vi "Build Command Frame.vi"(0 "RFFE Extended Command in":refnum<class "RFFE Extended Command.lvclass">, 11 "error in (no error)":errorcluster) -> (4 "RFFE Extended Command out":refnum<class "RFFE Extended Command.lvclass">, 6 "Command Frame":u8[](array[numeric]), 15 "error out":errorcluster)   [LabVIEW 2018, in "MIPI RFFE API.lvlib" / "RFFE Extended Command.lvclass"]
uses:
  RFFE Extended Command.lvclass
  C:/Users/semoore/Projects/mipi-rffe-labview-oop/Command/RFFE Command.lvclass
  Command/RFFE Command.lvclass/RFFE Command.ctl
  Command/Get Slave Address.vi
  Command/Get Command Bits.vi
  Get Byte Count Field Width.vi
  MIPI RFFE API.lvlib
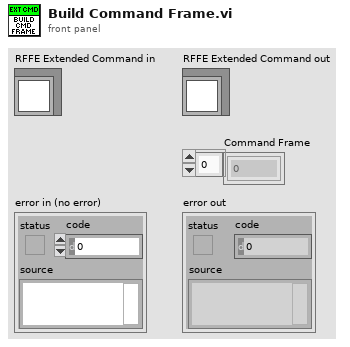
[diagram p1: front panel]
types:
  T1 = typedef "RFFE Commands.lvlib/Slave Address.ctl" = u8
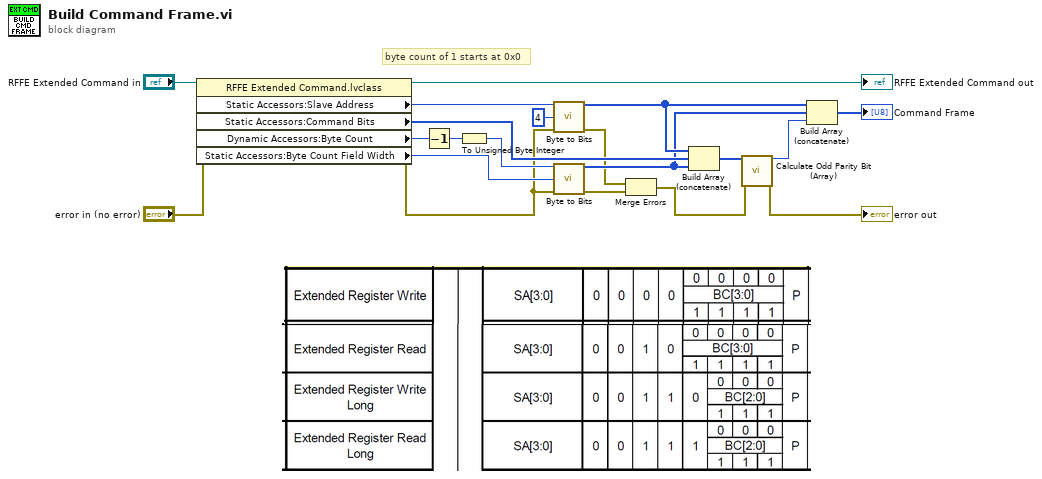
[diagram p0: block diagram]
diagram:
  # "byte count of 1 starts at 0x0"
  n1 = property class="RFFE Extended Command.lvclass"(reference="RFFE Extended Command in", error in="error in (no error)") -> (reference out=→"RFFE Extended Command out":refnum<class "RFFE Extended Command.lvclass">, error out=w6:errorcluster, "Static Accessors:Slave Address"=w9:T1, "Static Accessors:Command Bits"=w8:u8[], "Dynamic Accessors:Byte Count"=w1:i32, "Static Accessors:Byte Count Field Width"=w14:i32)
  n2 = Decrement(x=w1) -> (x-1=w2:i32)
  n3 = To Unsigned Byte Integer(number=w2) -> (unsigned 8bit integer=w13:u8)
  n4 = call "Byte to Bits.vi"("Byte"=w9, "Bit Width"=4, "error in (no error)"=w6) -> ("Bits"=w10:u8[], "error out"=w5:errorcluster)  [unwired: 11 in]
  n5 = call "Byte to Bits.vi"("Byte"=w13, "Bit Width"=w14, "error in (no error)"=w6) -> ("Bits"=w7:u8[], "error out"=w4:errorcluster)  [unwired: 11 in]
  n6 = Merge Errors(w5, w4) -> (w3:errorcluster)
  n7 = Build Array (concatenate)(w10, w8, w7) -> (w12:u8[])
  n8 = call "Calculate Odd Parity Bit (Array).vi"("Bytes"=w12, "error in (no error)"=w3) -> ("Odd Parity Bit"=w11:u8, "error out"=→"error out":errorcluster)  [unwired: 12 in]
  n9 = Build Array (concatenate)(w10, w7, w11) -> (→"Command Frame":u8[])
